vi "GetProfile Params.vi"(6 "Step (-1)":i32=-1, 7 "Steps from 0 (T)":bool=TRUE, 8 "error in (no error)":errorcluster, 10 "NO":u8=1 min=1 max=50 step=1, 11 "Application":T1) -> (0 "error out":errorcluster, 2 "wchitch params":string, 3 "params array out":string[](array[string]))   [LabVIEW 2021, in "STAV lib.lvlib"]
uses:
  STAV lib.lvlib
  Application.ctl
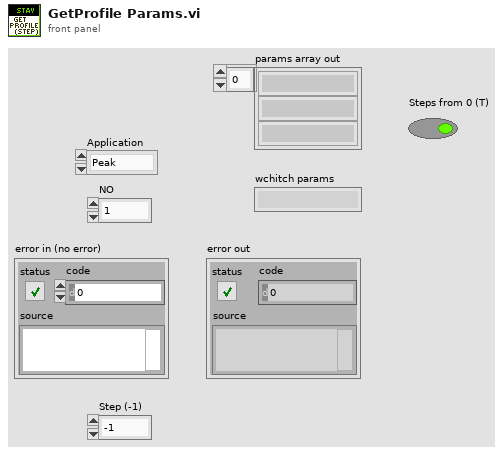
[diagram p1: front panel]
types:
  T1 = typedef "STAV lib.lvlib/Application.ctl" = enum16{"Peak", "Cycle", "Step", "Advanced"}
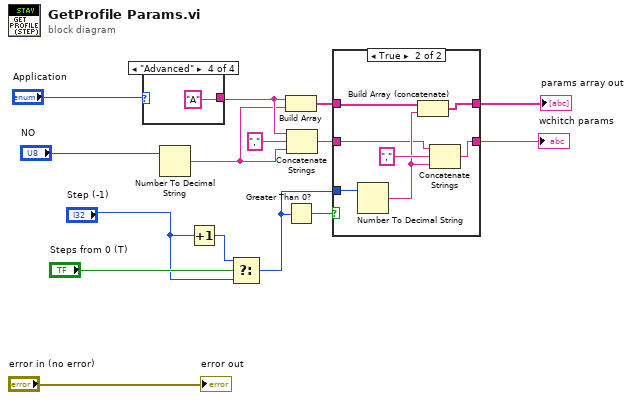
[diagram p0: block diagram]
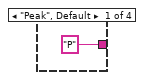
[diagram p3: hidden frame]
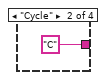
[diagram p4: hidden frame]
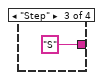
[diagram p5: hidden frame]
diagram:
  n1 = case shown="\"Advanced\"" "Application" {
    tunnel: ["P" "C" "S" "A"] -> w13
    frame "Peak", Default {
    }
    frame "Cycle" {
    }
    frame "Step" {
    }
    frame "Advanced" {
    }
  }
  n2 = Number To Decimal String(number="NO") -> (decimal integer string=w10:string)  [unwired: 1 in]
  n3 = Increment(x="Step (-1)") -> (x+1=w1:i32)
  n4 = Select(t=w1, s="Steps from 0 (T)", f="Step (-1)") -> (s? t:f=w3:i32)
  n5 = Build Array(w13, w10) -> (w7:string[])
  n6 = Greater Than 0?(x=w3) -> (x > 0?=w9:bool)
  n7 = Concatenate Strings(w13, "," ("string"), w10) -> (w8:string)
  n8 = case shown="True" w9 {
    tunnel: w8 -> [w20 w23]
    tunnel: w7 -> [w21 w27]
    tunnel: [w21 w26] -> w6
    tunnel: [w20 w22] -> w5
    tunnel: w3 -> [_ w28]
    frame False {
    }
    frame True {
      n9 = Number To Decimal String(number=w28) -> (decimal integer string=w24:string)  [unwired: 1 in]
      n10 = Build Array (concatenate)(w27, w24) -> (w26:string[])
      n11 = Concatenate Strings(w23, "," ("string"), w24) -> (w22:string)
    }
  }
  "params array out" <- w6
  "wchitch params" <- w5
  "error out" <- "error in (no error)"
